vi "ConvertTraceFormatElementsToItemList.vi"(11 "Trace Format Elements":T1[](array[typedef])) -> (3 "Item List":string)   [LabVIEW 8.6, in "Keithley-6482-Visa.lvlib"]
uses:
  Keithley-6482-Visa.lvlib
  Public/Controls/TraceFormatElement.ctl
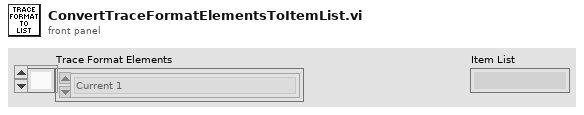
[diagram p1: front panel]
types:
  T1 = typedef "Keithley-6482-Visa.lvlib/TraceFormatElement.ctl" = enum16{"Current 1", "Current 2", "Calculate 1", "Calculate 2", "Calculate 3", "Calculate 4", "Calculate 5", "Calculate 6", "Calculate 7", "Time", "Status", "All", "Default"}
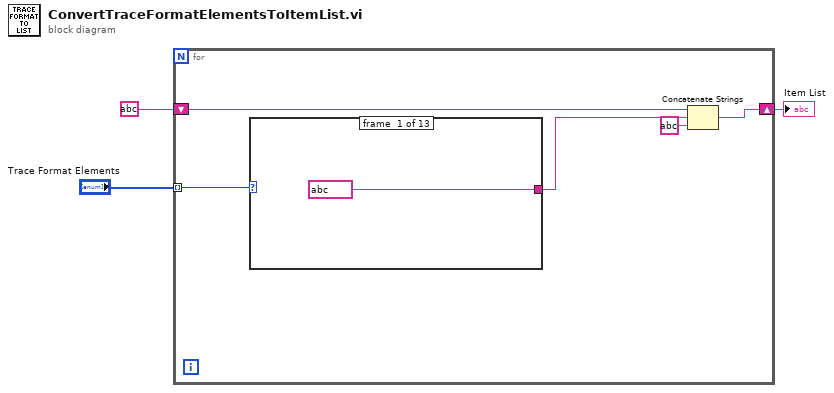
[diagram p0: block diagram]
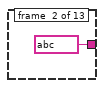
[diagram p2: hidden frame]
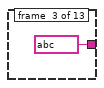
[diagram p3: hidden frame]
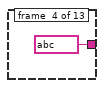
[diagram p4: hidden frame]
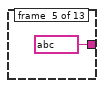
[diagram p5: hidden frame]
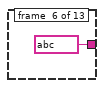
[diagram p6: hidden frame]
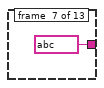
[diagram p7: hidden frame]
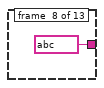
[diagram p8: hidden frame]
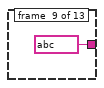
[diagram p9: hidden frame]
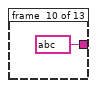
[diagram p10: hidden frame]
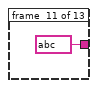
[diagram p11: hidden frame]
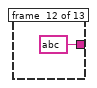
[diagram p12: hidden frame]
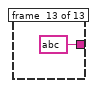
[diagram p13: hidden frame]
diagram:
  n1 = for {
    tunnel: "Trace Format Elements" -> [w6] mode=indexing
    shift-right: [w7] -> w1
    shift-left: string ? -> [w8]
    n2 = case shown="\"Default\"" w6 {
      tunnel: [string ? string ? string ? string ? string ? string ? string ? string ? string ? string ? string ? string ? string ?] -> w5
      frame #0 {
      }
      frame #1 {
      }
      frame #2 {
      }
      frame #3 {
      }
      frame #4 {
      }
      frame #5 {
      }
      frame #6 {
      }
      frame #7 {
      }
      frame #8 {
      }
      frame #9 {
      }
      frame #10 {
      }
      frame #11 {
      }
      frame #12 {
      }
    }
    n3 = Concatenate Strings(w8, w5, string ? ("string")) -> (w7:string)
  }
  "Item List" <- w1
